vi "waitForIRQ.vi"(8 "error in (no error)":errorcluster, 9 "Timeout (ms)":i32, 10 "IRQs in":i32[](array[numeric]), 11 "FPGA in":refnum<class "FPGA.lvclass">) -> (0 "error out":errorcluster, 1 "TimedOut":bool, 2 "IRQs out":i32[](array[numeric]), 3 "FPGA out":refnum<class "FPGA.lvclass">)   [LabVIEW 2016, in "FPGA.lvclass"]
uses:
  FPGA.lvclass
  FPGA.lvclass/FPGA.ctl
  <vilib>/Utility/error.llb/Error Cluster From Error Code.vi
  <vilib>/RVI Host/nirviSupport.llb/nirviErrorClusterFromErrorCode.vi
  <vilib>/rvi/errors/niLvFpgaAdjustHostInterfaceError.vi
  <vilib>/rvi/interface/nirviMethod/nirviMethod.xnode
  <vilib>/rvi/interface/nirviMethod/StockFPGA_InlinedMethodWaitForMultipleIRQ.vi
  <vilib>/FPGAPlugInAG/Dynamic/niLvFpga_WaitOnIrq_Dynamic.vi
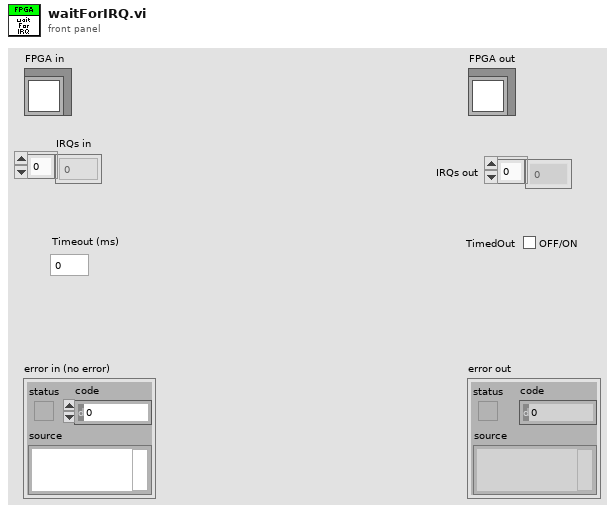
[diagram p1: front panel]
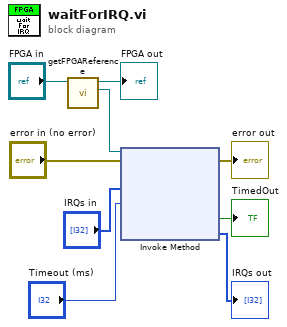
[diagram p0: block diagram]
diagram:
  n1 = call "getFPGAReference.vi"("FPGA in"="FPGA in") -> ("FPGAReference"=w8:refnum<k20>, "FPGA out"=→"FPGA out":refnum<class "FPGA.lvclass">)  [unwired: 9 in]
  n2 = xnode "Invoke Method"("FPGA VI Reference In"=w8, "error in"="error in (no error)", "IRQ Number(s)"="IRQs in", "Timeout (ms)"="Timeout (ms)") -> ("error out"=→"error out":errorcluster, "Timed Out"=→"TimedOut":bool, "IRQ(s) Asserted"=→"IRQs out":i32[])  [unwired: 1 out]
